vi "Show and Analyze.vi"(0 "Display State In":T3 {"Centroid"."Y Centroid" format="%.2f"; "Centroid"."X Centroid" format="%.2f"; "ROI"."Contours"."Type" items=["No Selection", "Point", "Line", "Rectangle", "Oval", "Polygon", "Freehand Region", "Annulus", "Unused2", "Unused3", "Broken Line", "Freehand Line", "Rotated Rectangle"]}, 5 "Image In":T1, 9 "Container State":T7, 11 "error in (no error)":errorcluster) -> (3 "Analysis Params":variant, 4 "Display State Out":T3 {"Centroid"."Y Centroid" format="%.2f"; "Centroid"."X Centroid" format="%.2f"; "ROI"."Contours"."Type" items=["No Selection", "Point", "Line", "Rectangle", "Oval", "Polygon", "Freehand Region", "Annulus", "Unused2", "Unused3", "Broken Line", "Freehand Line", "Rotated Rectangle"]}, 6 "Displayd Image":T1, 8 "ROI":T2 {"Contours"."Type" items=["No Selection", "Point", "Line", "Rectangle", "Oval", "Polygon", "Freehand Region", "Annulus", "Unused2", "Unused3", "Broken Line", "Freehand Line", "Rotated Rectangle"]}, 10 "calibr":sgl, 13 "elapsed ms":u32, 14 "Analysis Results":variant, 15 "error out":errorcluster)   [LabVIEW 2009, in "POLARIS IMAQ Display.xctl"]
uses:
  POLARIS IMAQ Display.xctl
  <vilib>/_xctls/Container State.ctl
  State.ctl
  IMAQdx Cam/IMAQdx Cam.lvclass
  Properties/ImageSource.ctl
  <vilib>/vision/Image Controls.llb/IMAQ Image.ctl
  DisplaySettings.ctl
  Named ROI.ctl
  Analyze Classes/Analyze BaseClass/Analyze BaseClass.lvclass
  Palette.ctl
  <vilib>/vision/NI_Vision_Development_Module.lvlib
  <vilib>/_xctls/XControlSupport.lvlib
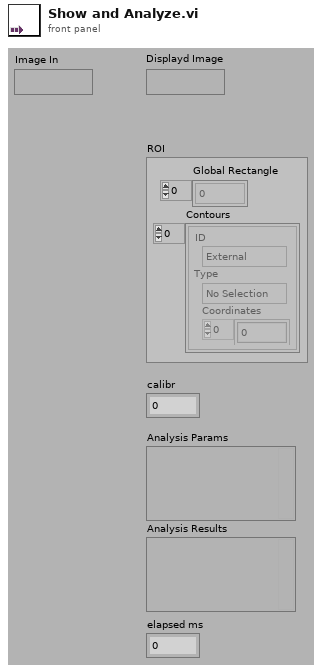
[diagram p1: front panel]
types:
  T1 = typedef "IMAQ Image.ctl" = refnum<image>
  T2 = typedef "ROI Descriptor" = cluster{"Global Rectangle":i32[], "Contours":cluster{"ID":enum32{"External", "Internal"}, "Type":u32, "Coordinates":i32[]}[]}
  T3 = typedef "POLARIS IMAQ Display.xctl/State.ctl" = cluster{"ImageSource":T4, "IMAQdx Cam":refnum<class "IMAQdx Cam.lvclass">, "WorkDir":path, "Image Name Prefix":string, "ROI":T2, "BG Image":T1, "Display Image":T1, "Display settings":T5, "Mask image":T1, "ConfigDir":path, "Display ref":refnum<vi>, "Saved ROIs":T6[], "Selected ROI":string, "Analyze Objects":refnum<class "Analyze BaseClass.lvclass">[], "Analysis Params":variant, "Analysis Results":variant, "Overlays?":bool[], "Ref Palette type":refnum<vi>, "Time in Filename?":bool, "Save Report?":bool, "Appl Params":variant, "Show ZoomBtn?":bool, "Image file":path, "SubstractBG?":bool, "Centroid":cluster{"X Centroid":sgl, "Y Centroid":sgl}, "Image In":T1}
  T4 = typedef "POLARIS IMAQ Display.xctl/ImageSource.ctl" = enum16{"Camera", "File"}
  T5 = typedef "POLARIS IMAQ Display.xctl/DisplaySettings.ctl" = cluster{"Min. Thresh.":sgl, "X":dbl, "Y":dbl, "ShowLineout":bool, "ScaleParts":i32, "ShowLegende":bool, "Target Cross":bool, "Centroid Cross":bool, "Target color":u32, "Centroid color":u32, "calibr. mm/px":sgl}
  T6 = typedef "POLARIS IMAQ Display.xctl/Named ROI.ctl" = cluster{"ROI":cluster{"Global Rectangle":i32[], "Contours":cluster{"Contour Type":u32, "ROI Type":u32, "Points":i32[]}[]}, "Name":string}
  T7 = typedef "XControlSupport.lvlib/Container State.ctl" = cluster{"Indicator?":bool, "Run Mode?":bool, " Refnum":refnum<vi>}
  T8 = typedef "Image Type" = u32
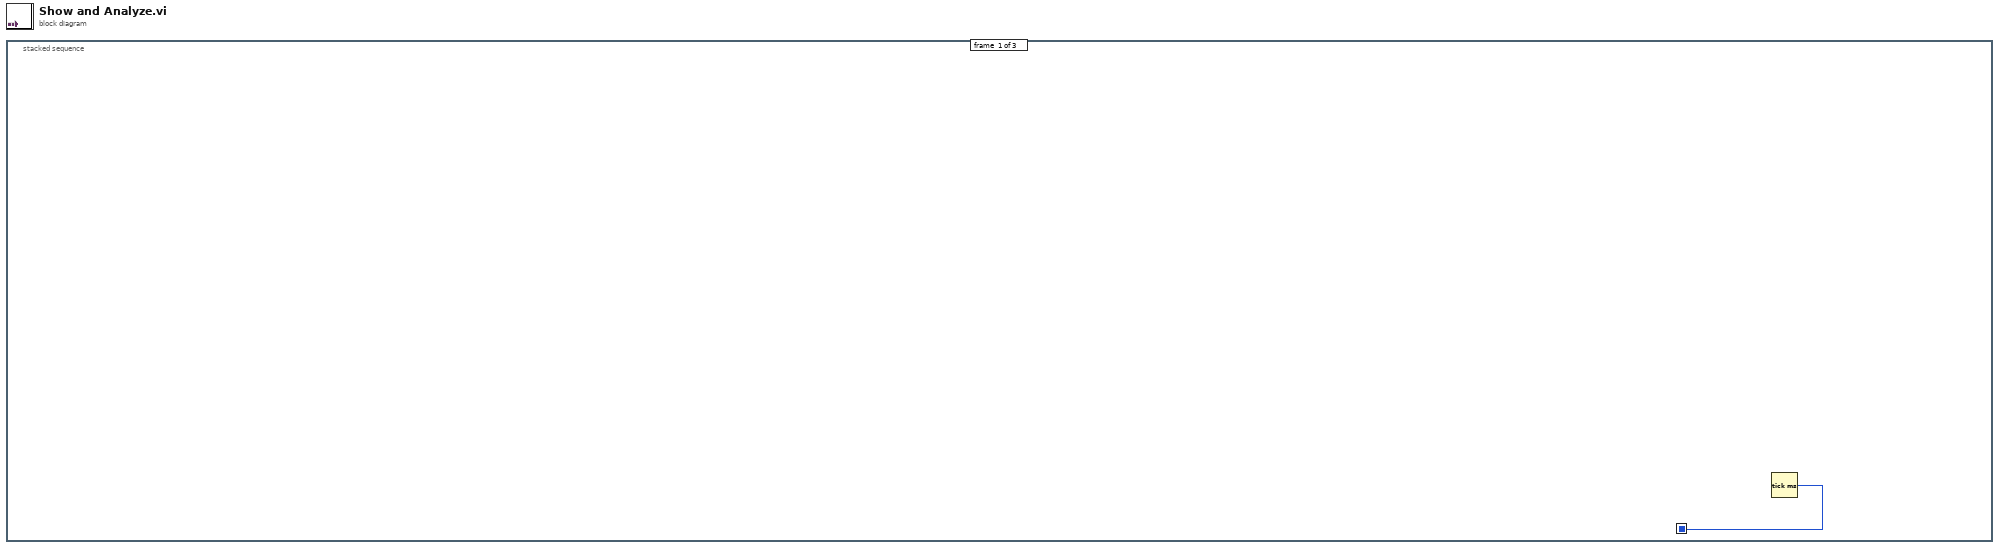
[diagram p0: block diagram]
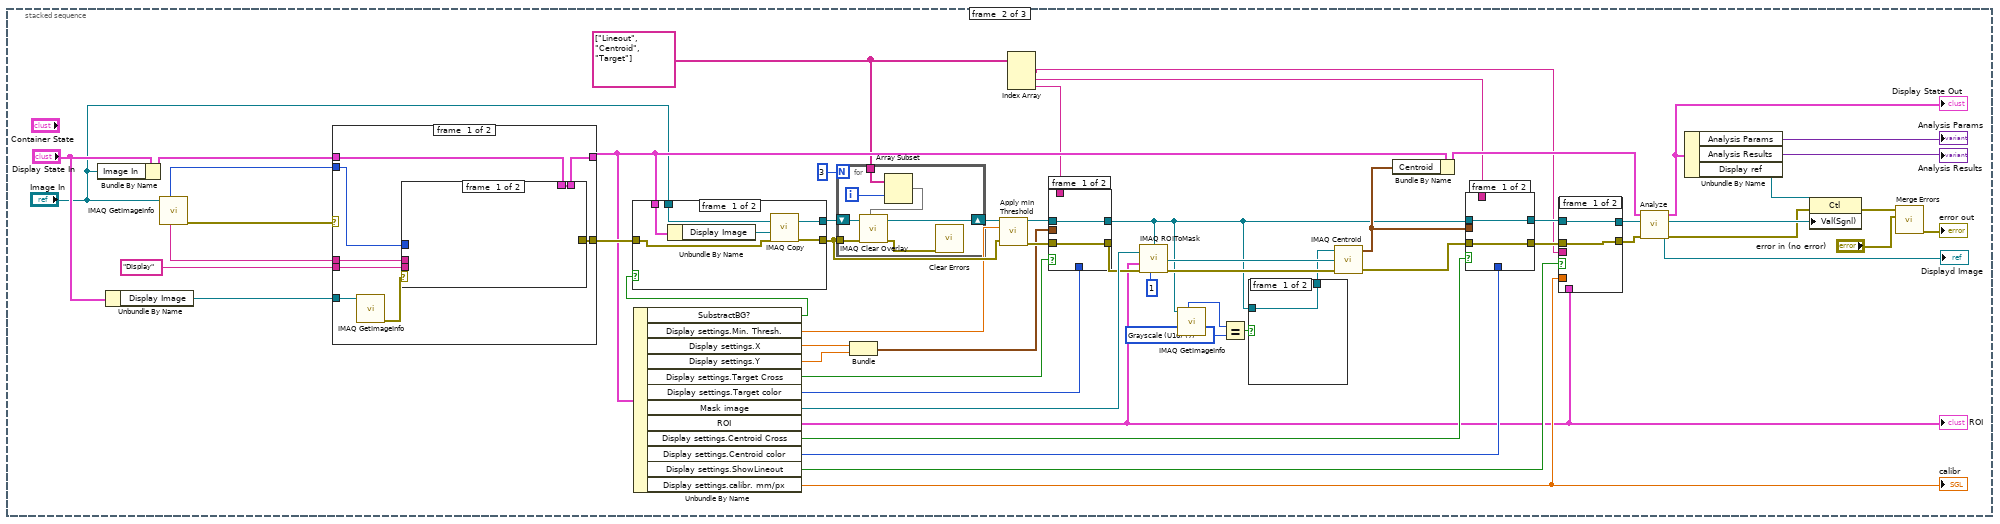
[diagram p2: hidden frame]
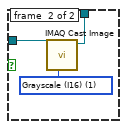
[diagram p3: hidden frame]
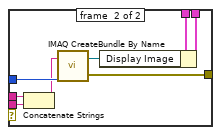
[diagram p4: hidden frame]
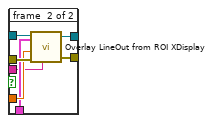
[diagram p6: hidden frame]
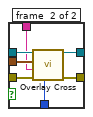
[diagram p7: hidden frame]
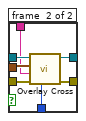
[diagram p8: hidden frame]
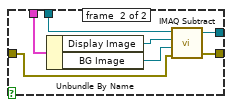
[diagram p9: hidden frame]
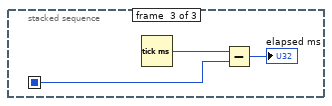
[diagram p10: hidden frame]
diagram:
  n1 = stacked-sequence {
    seq-local: [w1 _ _] -> [_ _ w132]
    frame #0 {
      n2 = Tick Count (ms)() -> (millisecond timer value=w1:u32)
    }
    frame #1 {
      w6 = T8 7 items=["Grayscale (U8)", "Grayscale (I16)", "Grayscale (SGL)", "Complex (CSG)", "RGB (U32)", "HSL (U32)", "RGB (U64)", "Grayscale (U16)"] ("Image Type")
      w10 = string[] ["Lineout", "Centroid", "Target"]
      n3 = Bundle By Name(cluster="Display State In", "Image In"="Image In") -> (w8:T3)
      n4 = Unbundle By Name("Display State In") -> ("Display Image"=w30:T1)
      n5 = call "IMAQ GetImageInfo"("Image"="Image In") -> ("error out"=w36:errorcluster, "Image Name"=w38:string, "Image Type"=w37:T8)  [unwired: 3 in, 5 out]
      n6 = case shown="No Error" w36 {
        selector: w36 -> [_ w88]
        tunnel: w8 -> [w78 w89]
        tunnel: [w77 w89] -> w28
        tunnel: [w76 w88] -> w39
        tunnel: w38 -> [w75 _]
        tunnel: w37 -> [w71 _]
        tunnel: "Display" ("string") -> [w74 _]
        tunnel: w30 -> [w73 _]
        frame #0 {
          n7 = call "IMAQ GetImageInfo"("Image"=w73) -> ("error out"=w72:errorcluster)  [unwired: 3 in, 7 out]
          n8 = case shown="Error" w72 {
            tunnel: w78 -> [w79 w87]
            tunnel: [w79 w86] -> w77
            tunnel: [_ w85] -> w76
            tunnel: w75 -> [_ w84]
            tunnel: w71 -> [_ w83]
            tunnel: w74 -> [_ w80]
            frame #0 {
            }
            frame #1 {
              n9 = Concatenate Strings(w84, w80) -> (w82:string)
              n10 = call "IMAQ Create"("Image Name"=w82, "Image Type"=w83) -> ("New Image"=w81:T1, "error out"=w85:errorcluster)  [unwired: 3 in]
              n11 = Bundle By Name(cluster=w87, "Display Image"=w81) -> (w86:T3)
            }
          }
        }
        frame #1 {
        }
      }
      n12 = Unbundle By Name(w28) -> ("SubstractBG?"=w9:bool, "Display settings.Min. Thresh."=w31:sgl, "Display settings.X"=w57:dbl, "Display settings.Y"=w56:dbl, "Display settings.Target Cross"=w55:bool, "Display settings.Target color"=w53:u32, "Mask image"=w49:T1, "ROI"=w26:T2, "Display settings.Centroid Cross"=w48:bool, "Display settings.Centroid color"=w45:u32, "Display settings.ShowLineout"=w42:bool, "Display settings.calibr. mm/px"=w27:sgl)
      "calibr" <- w27
      "ROI" <- w26
      n13 = case shown="False" w9 {
        tunnel: w28 -> [w122 w129]
        tunnel: "Image In" -> [w121 w126]
        tunnel: [w119 w127] -> w41
        tunnel: [w118 w124] -> w34
        tunnel: w39 -> [w117 w123]
        frame #0 {
          n14 = Unbundle By Name(w122) -> ("Display Image"=w120:T1)
          n15 = call "IMAQ Copy"("error in (no error)"=w117, "Image Dst"=w120, "Image Src"=w121) -> ("error out"=w118:errorcluster, "Image Dst Out"=w119:T1)  [unwired: 3 in]
        }
        frame #1 {
          n16 = Unbundle By Name(w129) -> ("Display Image"=w125:T1, "BG Image"=w128:T1)
          n17 = call "IMAQ Subtract"("Image Src A"=w126, "Image Dst"=w125, "Image Src B"=w128, "error in (no error)"=w123) -> ("Image Dst Out"=w127:T1, "error out"=w124:errorcluster)  [unwired: 3 in]
        }
      }
      n18 = for {
        N: 3 -> [_]
        tunnel: w34 -> [w68]
        shift-right: [w69] -> w40
        shift-left: w41 -> [w70]
        tunnel: w10 -> [w66]
        i -> [w65]
        n19 = Array Subset(array=w66, index=w65) -> (w64:string[])  [unwired: 1 in]
        n20 = call "IMAQ Clear Overlay"("Groups"=w64, "error in (no error)"=w68, "Image"=w70) -> ("error out"=w67:errorcluster, "Image Out"=w69:T1)  [unwired: 7 in]
        n21 = call <vilib>:"Clear Errors.vi"("error in (no error)"=w67) -> ()  [unwired: 6 in, 1 out]
      }
      n22 = Bundle("X"=w57, "Y"=w56) -> (w54:cluster{"X":dbl, "Y":dbl})  [unwired: 1 in]
      n23 = call "Apply min Threshold.vi"("error in"=w34, "Min. Thresh."=w31, "Image In"=w40) -> ("error out"=w58:errorcluster, "Image Out"=w59:T1)  [unwired: 7 in]
      n24 = Index Array(array=w10) -> (element #1=w14:string, element #2=w13:string, element #3=w12:string)  [unwired: 3 in]
      n25 = case shown="True" w55 {
        tunnel: w59 -> [w109 w116]
        tunnel: [w109 w115] -> w3
        tunnel: w58 -> [w108 w114]
        tunnel: w54 -> [_ w113]
        tunnel: w53 -> [_ w112]
        tunnel: [w108 w111] -> w47
        tunnel: w12 -> [_ w110]
        frame #0 {
        }
        frame #1 {
          n26 = call "Overlay Cross.vi"("Color"=w112, "error in (no error)"=w114, "Overlay Group"=w110, "point"=w113, "Image In"=w116) -> ("error out"=w111:errorcluster, "Image Out"=w115:T1)  [unwired: 4 in]
        }
      }
      n27 = call "IMAQ ROIToMask"("error in (no error)"=w47, "ROI Descriptor"=w26, "Filling Value (255)"=1, "Image"=w49, "Image Model"=w3) -> ("error out"=w52:errorcluster, "Image Out"=w51:T1)  [unwired: 1 in, 1 out]
      n28 = call "IMAQ GetImageInfo"("Image"=w3) -> ("Image Type"=w5:T8)  [unwired: 3 in, 7 out]
      n29 = Equal?(x=w5, y=w6) -> (x = y?=w4:bool)
      n30 = case shown="True" w4 {
        tunnel: w3 -> [w60 w63]
        tunnel: [w60 w61] -> w2
        frame #0 {
        }
        frame #1 {
          w62 = T8 1 items=["Grayscale (U8)", "Grayscale (I16)", "Grayscale (SGL)", "Complex (CSG)", "RGB (U32)", "HSL (U32)", "RGB (U64)", "Grayscale (U16)"] ("Image Type")
          n31 = call "IMAQ Cast Image"("Image Type"=w62, "Image Src"=w63) -> ("Image Dst Out"=w61:T1)  [unwired: 8 in, 1 out]
        }
      }
      n32 = call "IMAQ Centroid"("error in (no error)"=w52, "Image Mask"=w51, "Image"=w2) -> ("error out"=w46:errorcluster, "Centroid"=w19:cluster{"X Centroid":sgl, "Y Centroid":sgl})  [unwired: 1 in]
      n33 = Bundle By Name(cluster=w28, "Centroid"=w19) -> (w20:T3)
      n34 = case shown="True" w48 {
        tunnel: w3 -> [w100 w107]
        tunnel: [w100 w106] -> w44
        tunnel: w46 -> [w99 w105]
        tunnel: w19 -> [_ w104]
        tunnel: w45 -> [_ w103]
        tunnel: [w99 w102] -> w43
        tunnel: w13 -> [_ w101]
        frame #0 {
        }
        frame #1 {
          n35 = call "Overlay Cross.vi"("Color"=w103, "error in (no error)"=w105, "Overlay Group"=w101, "point"=w104, "Image In"=w107) -> ("error out"=w102:errorcluster, "Image Out"=w106:T1)  [unwired: 4 in]
        }
      }
      n36 = case shown="True" w42 {
        tunnel: w44 -> [w91 w98]
        tunnel: w43 -> [w90 w97]
        tunnel: [w91 w96] -> w33
        tunnel: [w90 w95] -> w32
        tunnel: w27 -> [_ w94]
        tunnel: w26 -> [_ w93]
        tunnel: w14 -> [_ w92]
        frame #0 {
        }
        frame #1 {
          n37 = call "Overlay LineOut from ROI XDisplay.vi"("Image In"=w98, "ROI"=w93, "Calbration"=w94, "Group"=w92, "error in"=w97) -> ("Image Out"=w96:T1, "error out"=w95:errorcluster)  [unwired: 1 in, 1 out]
        }
      }
      n38 = call "Analyze.vi"("error in"=w32, "Image in"=w33, "State in"=w20) -> ("error out"=w18:errorcluster, "Image out"=w21:T1, "State out"=w25:T3)  [unwired: 6 in]
      "Display State Out" <- w25
      "Displayd Image" <- w21
      n39 = Unbundle By Name(w25) -> ("Analysis Params"=→"Analysis Params":variant, "Analysis Results"=→"Analysis Results":variant, "Display ref"=w22:refnum<vi>)
      n40 = property class="Ctl"(reference=w22, error in=w18, "Val(Sgnl)"=w21) -> (error out=w15:errorcluster)  [unwired: 1 out]
      n41 = call <vilib>:"Merge Errors.vi"("error in 2 (no error)"="error in (no error)", "error in 1 (no error)"=w15) -> ("error out"=→"error out":errorcluster)  [unwired: 5 in]
    }
    frame #2 {
      n42 = Tick Count (ms)() -> (millisecond timer value=w131:u32)
      n43 = Subtract(x=w131, y=w132) -> (x-y=→"elapsed ms":u32)
    }
  }
